vi "Autosampler Wash Needle.vi"(7 "Correlation ID":u32, 8 "error in (no error)":errorcluster, 11 "Application in":refnum<class "Application.lvclass">) -> (0 "error out":errorcluster, 3 "Application out":refnum<class "Application.lvclass">)   [LabVIEW 2023, in "Application.lvlib" / "Application.lvclass"]
uses:
  Application.lvclass
  Application.lvclass/Application.ctl
  Hardware/Device Messages/Save CorrID Msg/Save CorrID Msg.lvclass/Save CorrID Msg.ctl
  <vilib>/ActorFramework/Message Enqueuer/Message Enqueuer.lvclass/Message Enqueuer.ctl
  <vilib>/ActorFramework/Message Enqueuer/Enqueue.vi
  Hardware/Device Messages/Save CorrID Msg/Save CorrID Msg.lvclass
  Hardware/Autosampler Messages/Wash Needle Msg/Wash Needle Msg.lvclass
  <vilib>/ActorFramework/Message Priority Queue/Priority Enqueue.vi
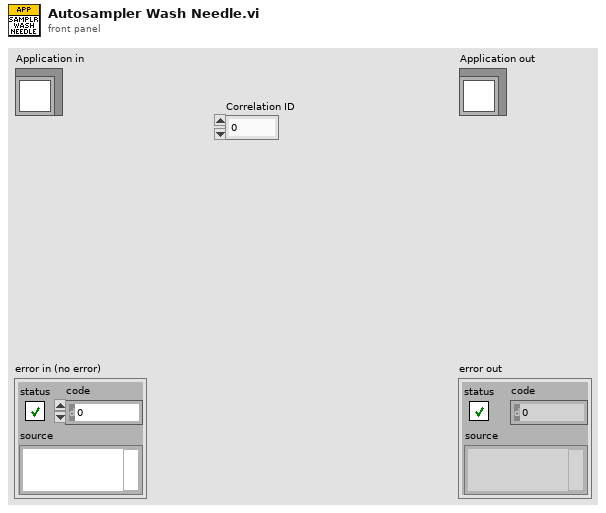
[diagram p1: front panel]
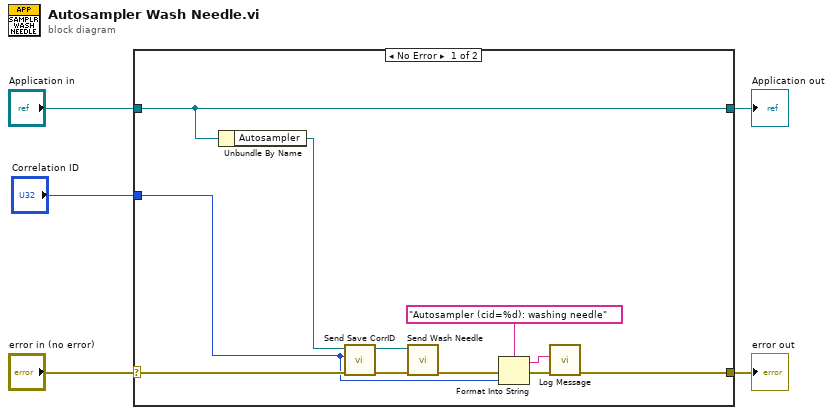
[diagram p0: block diagram]
diagram:
  n1 = case shown="No Error" "error in (no error)" {
    selector: "error in (no error)" -> [w14 w18]
    tunnel: [w15 w18] -> w4
    tunnel: [w16 w17] -> w2
    tunnel: "Application in" -> [w16 w17]
    tunnel: "Correlation ID" -> [w6 _]
    frame No Error {
      n2 = Unbundle By Name(w16) -> ("Autosampler"=w13:refnum<class "Message Enqueuer.lvclass">)
      n3 = call "Send Save CorrID.vi"("error in (no error)"=w14, "Correlation ID"=w6, "Message Enqueuer"=w13) -> ("error out"=w12:errorcluster, "Message Enqueuer out"=w11:refnum<class "Message Enqueuer.lvclass">)  [unwired: 7 in]
      n4 = call "Send Wash Needle.vi"("error in (no error)"=w12, "Message Enqueuer"=w11) -> ("error out"=w10:errorcluster)  [unwired: 8 in, 1 out]
      n5 = Format Into String(format string="Autosampler (cid=%d): washing needle", error in=w10, w6) -> (resulting string=w8:string, error out=w9:errorcluster)  [unwired: 1 in]
      n6 = call "Log Message.vi"("error constant"=w9, "input"=w8) -> ("error constant 2"=w15:errorcluster)  [unwired: 8 in, 1 out]
    }
    frame Error {
    }
  }
  "error out" <- w4
  "Application out" <- w2
